vi "ilcView.vi"() -> ()   [LabVIEW 2012]
uses:
  Typedefs/StateSelector.ctl
  CommandFactory/CommandFactory.lvclass
  State/ILCAppConfig.ctl
  Program Files (x86)/National Instruments/LabVIEW 2012/user.lib/Common/ILC/Configuration/ILCConfig.ctl
  Program Files (x86)/National Instruments/LabVIEW 2012/user.lib/Common/ILC/Configuration/InputChannels.ctl
  Program Files (x86)/National Instruments/LabVIEW 2012/user.lib/Common/ILC/Configuration/ScanRate_Hz_MultichannelOptions.ctl
  Program Files (x86)/National Instruments/LabVIEW 2012/user.lib/Common/SerialProtocols/Configuration/RS232Config.ctl
  Program Files (x86)/National Instruments/LabVIEW 2012/user.lib/Common/Component/Application/Configuration/ApplicationTiming.ctl
  UserEvents/UserEvents.lvclass
  UserEvents/UserEvents.lvclass/UserEvents.ctl
  Typedefs/CommandSelector.ctl
  <vilib>/Utility/error.llb/DialogType.ctl
  Commands/Start/Start.lvclass
  Commands/Start/Start.lvclass/Start.ctl
  Controller/controllerMain.vi
  Controller/Controller.lvclass
panel:
  out "Fault":string
  out "State:":T1
  in  "goToStandbyIsTrue":bool
  in  "clearErrorIsTrue":bool
  in  "exitIsTrue":bool
  in  "startIsTrue":bool
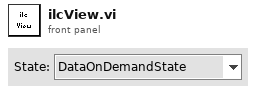
[diagram p1: front panel]
types:
  T1 = typedef "StateSelector.ctl" = enum16{"DataOnDemandState", "DataStreamingState", "FaultState", "OffState", "StandbyState"}
  T2 = typedef "ILCAppConfig.ctl" = cluster{"ILCConfig":T3, "RS232Config":T6, "Application Timing":T7}
  T3 = typedef "ILCConfig.ctl" = cluster{"Input Channels":T4, "Scan Rate (Hz) ":T5, "ADC PGA Gain":u8}
  T4 = typedef "InputChannels.ctl" = enum16{"Channel 0", "3 Channels", "5 Channels"}
  T5 = typedef "ScanRate_Hz_MultichannelOptions.ctl" = enum16{"50", "60", "100", "120", "200", "240", "300", "400", "480", "600", "1200", "2400", "4800"}
  T6 = typedef "RS232Config.ctl" = cluster{"VISA resource name":refnum<visa-resource-name>, "Baud Rate":u32, "Data Bits":u16, "Parity":enum16{"None", "Odd", "Even", "Mark", "Space"}, "Stop Bits":u16, "Flow Control":u16, "Timeout (ms)":u32}
  T7 = typedef "ApplicationTiming.ctl" = cluster{"Loop Period (ms)":u16}
  T8 = enum32{"invalid app kind", "Development System", "Run Time System", "Student Edition", "Embedded LabVIEW", "Evaluation", "Custom"}
  T9 = typedef "PubDataEvents.ctl" = cluster{"State":refnum<user-event>, "ErrorCode":refnum<user-event>, "OutputData":refnum<user-event>, "InputData":refnum<user-event>, "ILCConfig":refnum<user-event>, "NeedUserOutputs":refnum<user-event>}
  T10 = typedef "SubDataEvents.ctl" = cluster{"Command":refnum<user-event>}
  T11 = cluster{"Event Registration Refnum":refnum<event-registration>, "Event Registration Refnum":refnum<event-registration>}
  T12 = typedef "CommandSelector.ctl" = enum16{"ClearError", "Exit", "StandBy", "Start", "SwitchToOnDemandMode", "SwitchToStreamMode", "Update"}
  T13 = typedef "DialogType.ctl" = u16
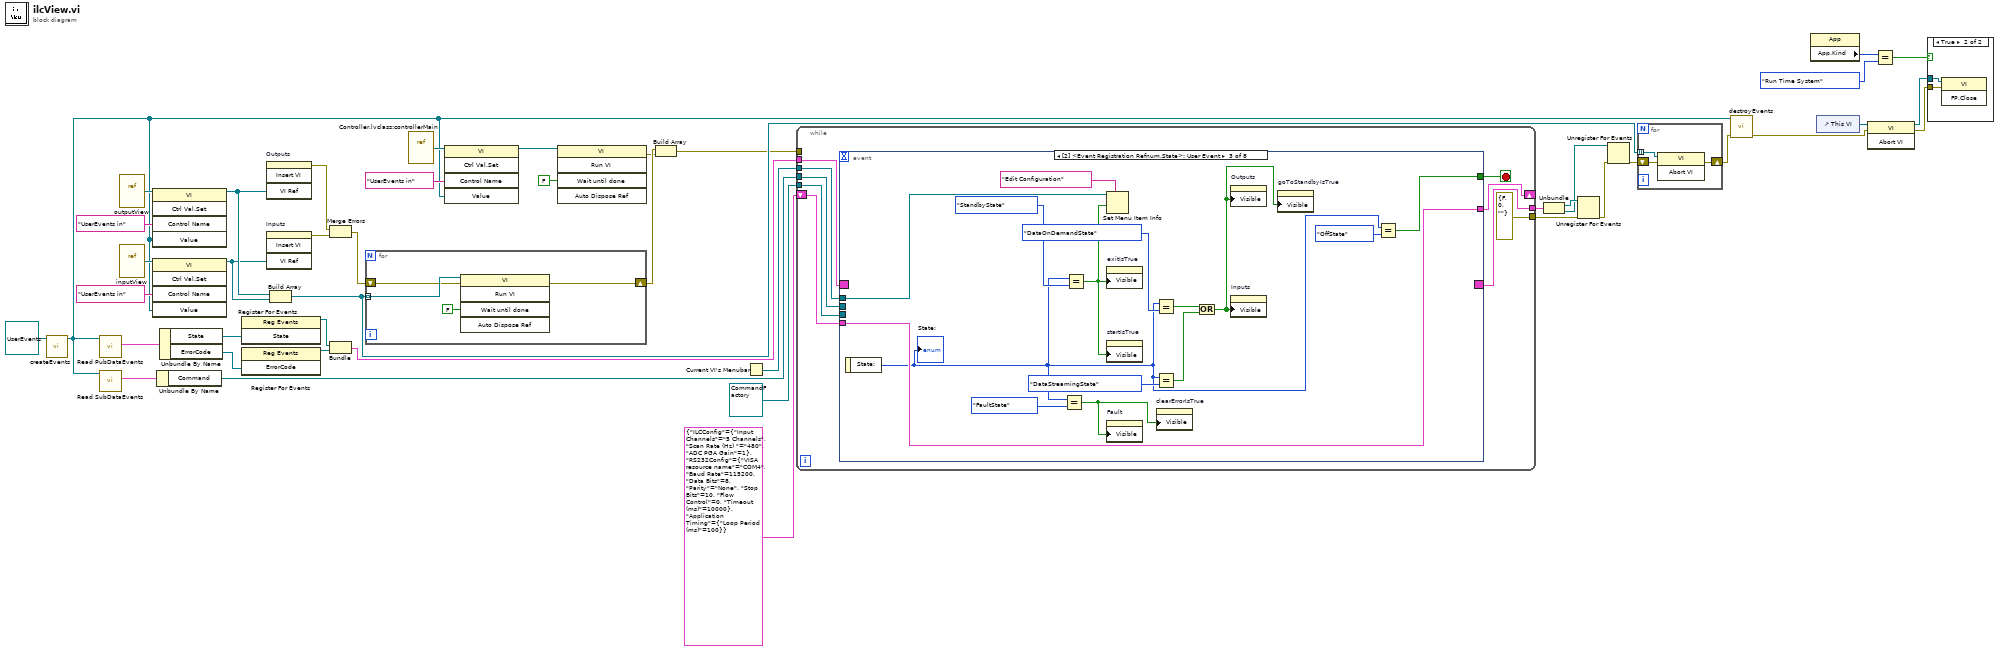
[diagram p0: block diagram]
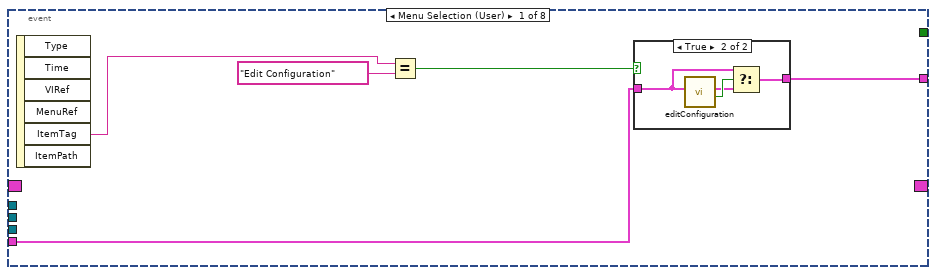
[diagram p3: hidden frame]
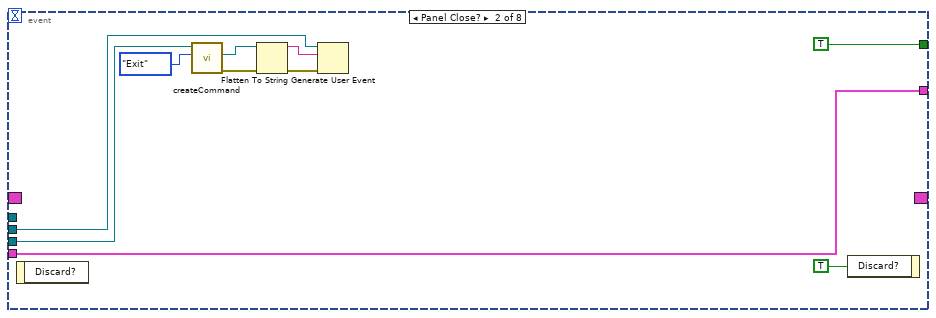
[diagram p5: hidden frame]
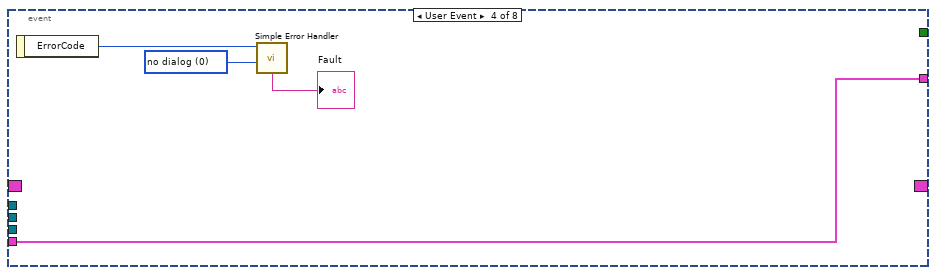
[diagram p6: hidden frame]
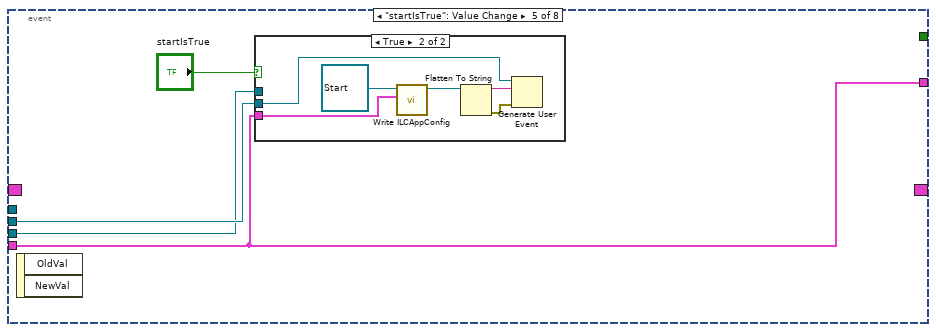
[diagram p7: hidden frame]
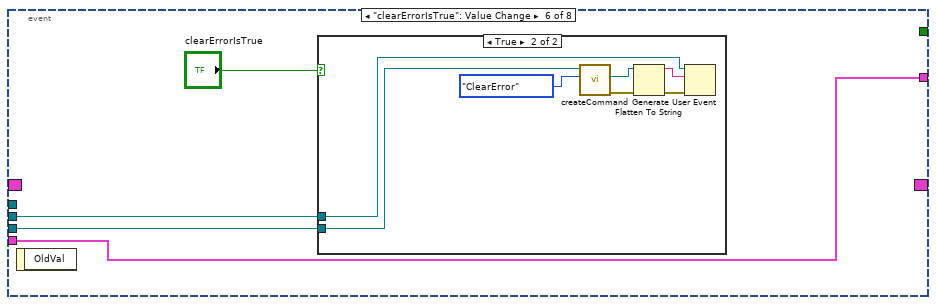
[diagram p9: hidden frame]
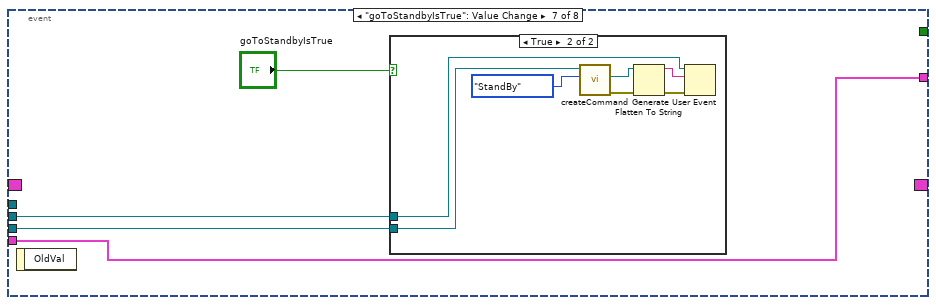
[diagram p11: hidden frame]
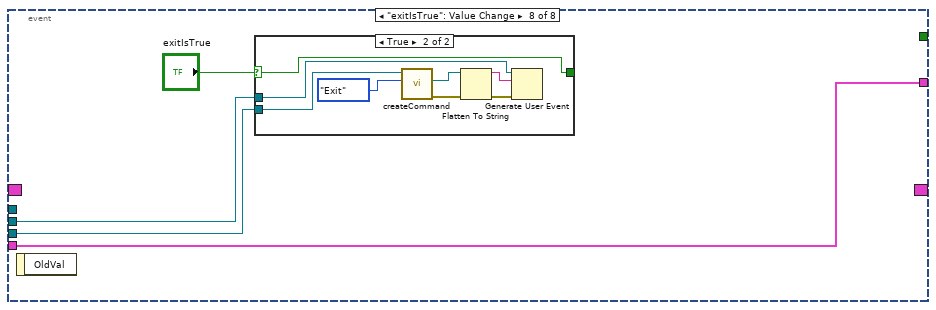
[diagram p13: hidden frame]
diagram:
  n1 = call "createEvents.vi"("UserEvents in"=refnum<class "UserEvents.lvclass"> refnum) -> ("UserEvents out"=w4:refnum<class "UserEvents.lvclass">)  [unwired: 9 in, 1 out]
  n2 = call "Read PubDataEvents.vi"("UserEvents in"=w4) -> ("PubDataEvents"=w31:T9)  [unwired: 9 in, 1 out]
  n3 = call "Read SubDataEvents.vi"("UserEvents in"=w4) -> ("SubDataEvents"=w29:T10)  [unwired: 9 in, 1 out]
  n4 = vi-ref "outputView.vi"() -> (w9:refnum<vi>)
  n5 = vi-ref "inputView.vi"() -> (w17:refnum<vi>)
  n6 = invoke class="VI" method="Ctrl Val.Set"(reference=w9, "Control Name"="UserEvents in", "Value"=w4) -> (reference out=w8:refnum<vi>)  [unwired: 2 in, 4 out]
  n7 = invoke class="VI" method="Ctrl Val.Set"(reference=w17, "Control Name"="UserEvents in", "Value"=w4) -> (reference out=w7:refnum<vi>)  [unwired: 2 in, 4 out]
  n8 = Unbundle By Name(w29) -> ("Command"=w28:refnum<user-event>)
  n9 = Unbundle By Name(w31) -> ("State"=w27:refnum<user-event>, "ErrorCode"=w25:refnum<user-event>)
  n10 = register-events(w27) -> (reference out=w26:refnum<event-registration>)  [unwired: 2 in, 1 out]
  n11 = register-events(w25) -> (reference out=w24:refnum<event-registration>)  [unwired: 2 in, 1 out]
  n12 = invoke on="Outputs" class="SubPanel" method="Insert VI"("VI Ref"=w8) -> (error out=w38:errorcluster)  [unwired: 3 in, 3 out]
  n13 = invoke on="Inputs" class="SubPnl" method="Insert VI"("VI Ref"=w7) -> (error out=w37:errorcluster)  [unwired: 3 in, 3 out]
  n14 = Build Array(w8, w7) -> (w35:refnum<vi>[])
  n15 = Merge Errors(w38, w37) -> (w36:errorcluster)
  n16 = Bundle("Event Registration Refnum"=w26, "Event Registration Refnum"=w24) -> (w15:T11)  [unwired: 1 in]
  n17 = for {
    tunnel: w35 -> [w48] mode=indexing
    shift-right: [w47] -> w3
    shift-left: w36 -> [w46]
    n18 = invoke class="VI" method="Run VI"(reference=w48, error in=w46, "Wait until done"=FALSE ("Wait Until Done")) -> (error out=w47:errorcluster)  [unwired: 2 in, 4 out]
  }
  n19 = vi-ref "Controller.lvclass:controllerMain.vi"() -> (w22:refnum<vi>)
  n20 = invoke class="VI" method="Ctrl Val.Set"(reference=w22, "Control Name"="UserEvents in", "Value"=w4) -> (reference out=w20:refnum<vi>)  [unwired: 2 in, 4 out]
  n21 = invoke class="VI" method="Run VI"(reference=w20, "Wait until done"=FALSE ("Wait Until Done")) -> (error out=w2:errorcluster)  [unwired: 3 in, 4 out]
  n22 = Build Array(w3, w2) -> (w1:errorcluster[])
  n23 = Current VI's Menubar() -> (w33:refnum<k9>)
  n24 = while {
    tunnel: refnum<class "CommandFactory.lvclass"> refnum ("CommandFactory.lvclass") -> [w54]
    tunnel: [errorcluster {"status"=FALSE, "code"=0, "source"=""} ("error out")] -> w16
    tunnel: w33 -> [w50]
    shift-right: [w53] -> _
    shift-left: T2 {"ILCConfig"={"Input Channels"=enum."5 Channels", "Scan Rate (Hz) "=enum."480", "ADC PGA Gain"=1}, "RS232Config"={"VISA resource name"="COM4", "Baud Rate"=115200, "Data Bits"=8, "Parity"=enum."None", "Stop Bits"=10, "Flow Control"=0, "Timeout (ms)"=10000}, "Application Timing"={"Loop Period (ms)"=100}} ("ILCAppConfig 2") -> [w52]
    tunnel: w15 -> [w56]
    tunnel: w28 -> [w51]
    tunnel: [w49] -> w14
    tunnel: w1 -> [_]
    stop <- w55 stop-if-true
    n25 = event shown="[2] <Event Registration Refnum.State>: User Event" {
      selector: w56 -> [_ _ _ _ _ _ _ _]
      dyn-events: [_ _ _ _ _ _ _ _] -> w49
      timeout: _ -> [_ _ _ _ _ _ _ _]
      tunnel: [_ TRUE w78 _ _ _ _ _] -> w55
      tunnel: w54 -> [_ w72 _ _ w98 w109 w120 w131]
      tunnel: [w59 w71 w81 w93 w97 w107 w118 w129] -> w53
      tunnel: w52 -> [w60 w71 w81 w93 w97 w107 w118 w129]
      tunnel: w51 -> [_ w68 _ _ w99 w108 w119 w130]
      tunnel: w50 -> [_ _ w82 _ _ _ _ _]
      event Menu Selection (User) {
        n26 = event-data() -> ("ItemTag"=w58:string)  [unwired: 1 in, 5 out]
        n27 = Equal?(x=w58, y="Edit Configuration") -> (x = y?=w62:bool)
        n28 = case shown="True" w62 {
          tunnel: [w63 w67] -> w59
          tunnel: w60 -> [w63 w65]
          frame False {
          }
          frame True {
            n29 = call "editConfiguration.vi"("ILCAppConfig"=w65) -> ("canceledIsTrue"=w66:bool, "ILCAppConfig 2"=w64:T2)  [unwired: 9 in]
            n30 = Select(t=w65, s=w66, f=w64) -> (s? t:f=w67:T2)
          }
        }
      }
      event Panel Close? {
        n31 = event-data() -> ()  [unwired: 1 in, 1 out]
        n32 = call-dynamic "createCommand.vi"("Command"=CommandSelector."Exit", "CommandFactory in"=w72) -> ("error out"=w77:errorcluster, "command"=w76:refnum<class "Command.lvclass">)  [unwired: 7 in, 1 out]
        n33 = Flatten To String(anything=w76, error in (no error)=w77) -> (data string=w69:string, error out=w70:errorcluster)  [unwired: 2 in, 1 out]
        n34 = Generate User Event(user event=w68, event data cluster=w69, error in=w70) -> ()  [unwired: 2 out]
        n35 = event-data("Discard?"=TRUE) -> ()  [unwired: 1 in, 1 out]
      }
      event User Event {
        n36 = event-data() -> ("State:"=w80:T1)  [unwired: 1 in]
        "State:" <- w80
        n37 = Equal?(x=w80, y=StateSelector."FaultState") -> (x = y?=w85:bool)
        n38 = Equal?(x=w80, y=StateSelector."StandbyState") -> (x = y?=w83:bool)
        n39 = Set Menu Item Info(7:"Edit Configuration" ("item name"), 9:w83, 11:w82) -> ()  [unwired: 4 in, 2 out]
        n40 = property on="exitIsTrue" class="Bool"("Visible"=w83) -> ()  [unwired: 2 in, 2 out]
        n41 = property on="startIsTrue" class="Bool"("Visible"=w83) -> ()  [unwired: 2 in, 2 out]
        n42 = property on="Fault" class="Str"("Visible"=w85) -> ()  [unwired: 2 in, 2 out]
        n43 = Equal?(x=w80, y=StateSelector."DataOnDemandState") -> (x = y?=w90:bool)
        n44 = Equal?(x=w80, y=StateSelector."DataStreamingState") -> (x = y?=w91:bool)
        n45 = property on="clearErrorIsTrue" class="Bool"("Visible"=w85) -> ()  [unwired: 2 in, 2 out]
        n46 = Or(x=w90, y=w91) -> (x .or. y?=w92:bool)
        n47 = property on="Outputs" class="SubPnl"("Visible"=w92) -> ()  [unwired: 2 in, 2 out]
        n48 = property on="Inputs" class="SubPnl"("Visible"=w92) -> ()  [unwired: 2 in, 2 out]
        n49 = property on="goToStandbyIsTrue" class="Bool"("Visible"=w92) -> ()  [unwired: 2 in, 2 out]
        n50 = Equal?(x=w80, y=StateSelector."OffState") -> (x = y?=w78:bool)
      }
      event User Event {
        w95 = T13 0 items=["no dialog", "OK message", "continue or stop message", "OK message + warnings", "continue/stop + warnings"] ("type of dialog (OK msg:1)")
        n51 = event-data() -> ("ErrorCode"=w94:i32)  [unwired: 1 in]
        n52 = call <vilib>:"Simple Error Handler.vi"("error code (no error:0)"=w94, "type of dialog (OK msg:1)"=w95) -> ("message"=→"Fault":string)  [unwired: 3 in, 4 out]
      }
      event "startIsTrue": Value Change {
        n53 = event-data() -> ()  [unwired: 1 in, 2 out]
        n54 = case shown="True" "startIsTrue" {
          tunnel: w99 -> [_ w104]
          tunnel: w98 -> [_ _]
          tunnel: w97 -> [_ w102]
          frame False {
          }
          frame True {
            n55 = call "Write ILCAppConfig.vi"("ILCAppConfig"=w102, "Start in"=refnum<class "Start.lvclass"> refnum ("Start.lvclass")) -> ("Start out"=w101:refnum<class "Start.lvclass">)  [unwired: 9 in]
            n56 = Flatten To String(anything=w101) -> (data string=w106:string, error out=w105:errorcluster)  [unwired: 3 in, 1 out]
            n57 = Generate User Event(user event=w104, event data cluster=w106, error in=w105) -> ()  [unwired: 2 out]
          }
        }
      }
      event "clearErrorIsTrue": Value Change {
        n58 = event-data() -> ()  [unwired: 1 in, 1 out]
        n59 = case shown="True" "clearErrorIsTrue" {
          tunnel: w109 -> [_ w117]
          tunnel: w108 -> [_ w111]
          frame False {
          }
          frame True {
            n60 = call-dynamic "createCommand.vi"("Command"=CommandSelector."ClearError", "CommandFactory in"=w117) -> ("error out"=w114:errorcluster, "command"=w115:refnum<class "Command.lvclass">)  [unwired: 7 in, 1 out]
            n61 = Flatten To String(anything=w115, error in (no error)=w114) -> (data string=w112:string, error out=w113:errorcluster)  [unwired: 2 in, 1 out]
            n62 = Generate User Event(user event=w111, event data cluster=w112, error in=w113) -> ()  [unwired: 2 out]
          }
        }
      }
      event "goToStandbyIsTrue": Value Change {
        n63 = event-data() -> ()  [unwired: 1 in, 1 out]
        n64 = case shown="True" "goToStandbyIsTrue" {
          tunnel: w120 -> [_ w128]
          tunnel: w119 -> [_ w122]
          frame False {
          }
          frame True {
            n65 = call-dynamic "createCommand.vi"("Command"=CommandSelector."StandBy", "CommandFactory in"=w128) -> ("error out"=w125:errorcluster, "command"=w126:refnum<class "Command.lvclass">)  [unwired: 7 in, 1 out]
            n66 = Flatten To String(anything=w126, error in (no error)=w125) -> (data string=w124:string, error out=w123:errorcluster)  [unwired: 2 in, 1 out]
            n67 = Generate User Event(user event=w122, event data cluster=w124, error in=w123) -> ()  [unwired: 2 out]
          }
        }
      }
      event "exitIsTrue": Value Change {
        n68 = event-data() -> ()  [unwired: 1 in, 1 out]
        n69 = case shown="True" "exitIsTrue" {
          selector: "exitIsTrue" -> [w133 w141]
          tunnel: [w133 w141] -> _
          tunnel: w131 -> [_ w140]
          tunnel: w130 -> [_ w134]
          frame False {
          }
          frame True {
            n70 = call-dynamic "createCommand.vi"("Command"=CommandSelector."Exit", "CommandFactory in"=w140) -> ("error out"=w137:errorcluster, "command"=w138:refnum<class "Command.lvclass">)  [unwired: 7 in, 1 out]
            n71 = Flatten To String(anything=w138, error in (no error)=w137) -> (data string=w135:string, error out=w136:errorcluster)  [unwired: 2 in, 1 out]
            n72 = Generate User Event(user event=w134, event data cluster=w135, error in=w136) -> ()  [unwired: 2 out]
          }
        }
      }
    }
  }
  n73 = Unbundle(w14) -> ("Event Registration Refnum"=w13:refnum<event-registration>, "Event Registration Refnum"=w11:refnum<event-registration>)
  n74 = Unregister For Events(event registration refnum=w13, error in=w16) -> (error out=w12:errorcluster)
  n75 = Unregister For Events(event registration refnum=w11, error in=w12) -> (error out=w10:errorcluster)
  n76 = for {
    tunnel: w35 -> [w144] mode=indexing
    shift-right: [w142] -> w6
    shift-left: w10 -> [w143]
    n77 = invoke class="VI" method="Abort VI"(reference=w144, error in=w143) -> (error out=w142:errorcluster)  [unwired: 1 in, 2 out]
  }
  n78 = call "destroyEvents.vi"("error in (no error)"=w6, "UserEvents in"=w4) -> ("error out"=w5:errorcluster)  [unwired: 8 in, 1 out]
  n79 = property class="App"() -> ("App.Kind"=w43:T8)  [unwired: 2 in, 2 out]
  n80 = control-ref of="This VI"() -> (w44:refnum<vi>)
  n81 = invoke class="VI" method="Abort VI"(reference=w44, error in=w5) -> (reference out=w41:refnum<vi>, error out=w40:errorcluster)  [unwired: 1 in, 1 out]
  n82 = Equal?(x=w43, y=T8."Run Time System") -> (x = y?=w39:bool)
  n83 = case shown="True" w39 {
    tunnel: w41 -> [_ w146]
    tunnel: w40 -> [_ w145]
    frame False {
    }
    frame True {
      n84 = invoke class="VI" method="FP.Close"(reference=w146, error in=w145) -> ()  [unwired: 1 in, 3 out]
    }
  }
